vi "Init FPGA code.vi"(8 "error in (no error)":errorcluster, 11 "Device Ref in":T1 format="%.0x") -> (0 "Error out":errorcluster, 1 "DMA FIFO ref":refnum<k20>, 2 "Bitfile ref":refnum<k20>, 3 "Device Ref out":T1 format="%.0x")   [LabVIEW 2014, in "SLSC configuration Engine.lvlib"]
uses:
  SLSC configuration Engine.lvlib
  <vilib>/NI Veristand/Custom Device API/Custom Device Item Ref.ctl
  <vilib>/NI Veristand/Custom Device API/Custom Device API.lvlib
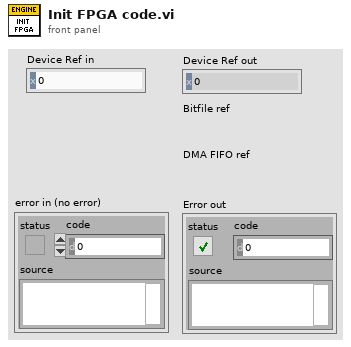
[diagram p1: front panel]
types:
  T1 = typedef "Custom Device API.lvlib/Custom Device Item Ref.ctl" = u64
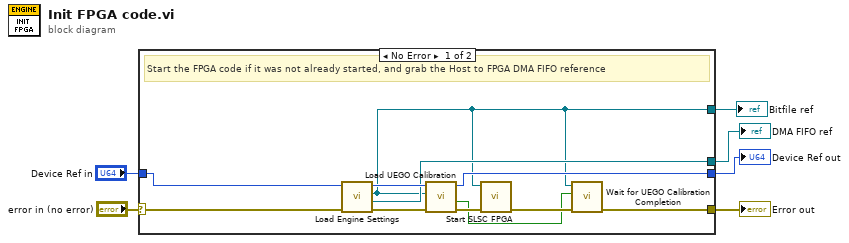
[diagram p0: block diagram]
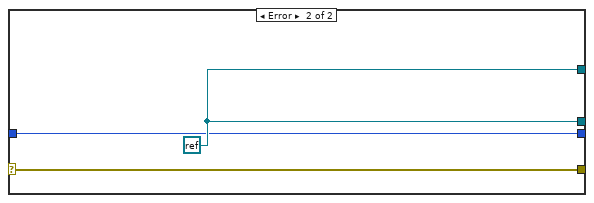
[diagram p2: hidden frame]
diagram:
  n1 = case shown="No Error" "error in (no error)" {
    selector: "error in (no error)" -> [w16 w19]
    tunnel: "Device Ref in" -> [w17 w18]
    tunnel: [w7 w20] -> w6
    tunnel: [w13 w20] -> w2
    tunnel: [w9 w19] -> w5
    tunnel: [w8 w18] -> w1
    frame No Error {
      # "Start the FPGA code if it was not already started, and grab the Host to FPGA DMA FIFO reference"
      n2 = call "Load Engine Settings.vi"("error in (no error)"=w16, "Device Ref in"=w17) -> ("error out"=w15:errorcluster, "FIFO Ref out"=w13:refnum<k20>, "FPGA Ref out"=w7:refnum<k20>, "Device Ref out"=w14:T1)  [unwired: 6 in]
      n3 = call "Load UEGO Calibration.vi"("error in (no error)"=w15, "FPGA Ref in"=w7, "Device Ref in"=w14) -> ("error out"=w12:errorcluster, "UEGO Present?"=w10:bool, "Device Ref out"=w8:T1)  [unwired: 6 in]
      n4 = call "Start SLSC FPGA.vi"("error in (no error)"=w12, "FPGA Ref in"=w7) -> ("error out"=w11:errorcluster)  [unwired: 9 in]
      n5 = call "Wait for UEGO Calibration Completion.vi"("error in"=w11, "UEGO Present?"=w10, "FPGA Ref in"=w7) -> ("error out"=w9:errorcluster)  [unwired: 8 in]
    }
    frame Error {
      w20 = refnum<k0> refnum
    }
  }
  "Bitfile ref" <- w6
  "Error out" <- w5
  "Device Ref out" <- w1
  "DMA FIFO ref" <- w2
